vi "SPI Regs.vi"() -> (0 "Init Data Out":u64[](array[numeric]))   [LabVIEW 2018]
panel:
  # "For Initialization VI requirements and help, please read directions located on Block Diagram."
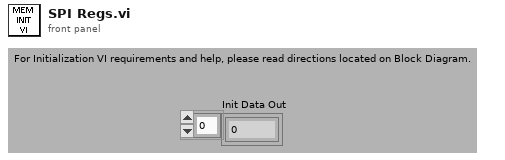
[diagram p1: front panel]
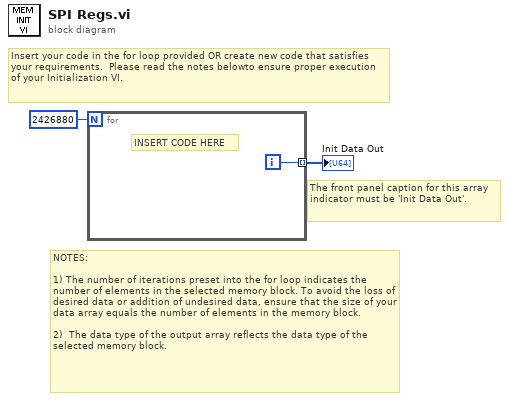
[diagram p0: block diagram]
diagram:
  # "The front panel caption for this array indicator must be 'Init Data Out'."
  # "NOTES:\n\n1) The number of iterations preset into the for loop indicates the number of elements in the selected memory block. To avoid the loss of desired data or addition of undesired data, ensure that the size of your data array equals the number of elements in the memory block.\n\n2)  The data type of the output array reflects the data type of the selected memory block."
  # "Insert your code in the for loop provided OR create new code that satisfies your requirements.  Please read the notes belowto ensure proper execution of your Initialization VI."
  n1 = for {
    N: 2426880 ("Number of Elements") -> [_]
    tunnel: [w3] -> w1 mode=indexing
    i -> [w3]
    # "INSERT CODE HERE"
  }
  "Init Data Out" <- w1
